vi "Auton Ramper.vi"(9 "Target Setpoint":dbl=3.01, 11 "Rate":dbl) -> (1 "Ramping":bool, 3 "Current Setpoint":dbl)   [LabVIEW 2011]
uses:
  Robot Global Data.vi
panel:
  out "crement":dbl
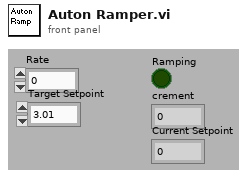
[diagram p1: front panel]
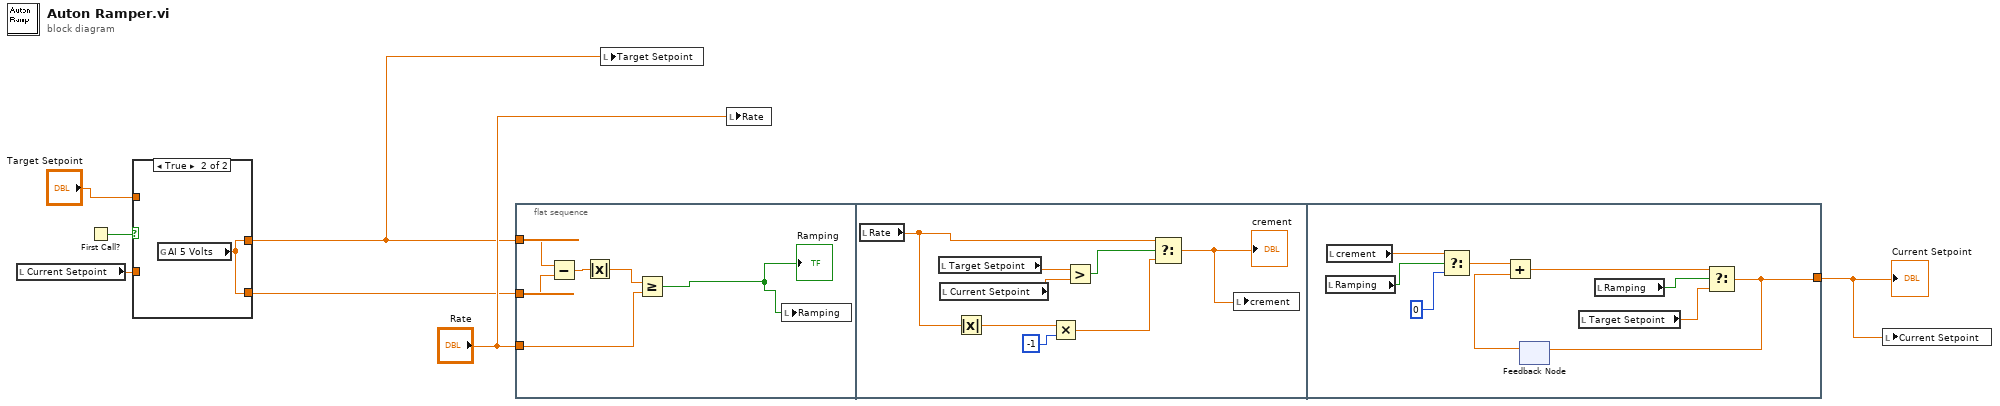
[diagram p0: block diagram]
diagram:
  n1 = local read "Current Setpoint"() -> (w4:dbl)
  n2 = First Call?() -> (First Call?: T/F=w3:bool)
  n3 = case shown="True" w3 {
    tunnel: "Target Setpoint" -> [w9 _]
    tunnel: w4 -> [w8 _]
    tunnel: [w9 w10] -> w2
    tunnel: [w8 w10] -> w1
    frame False {
    }
    frame True {
      n4 = global read "Robot Global Data.vi" "AI 5 Volts"() -> (w10:dbl)
    }
  }
  n5 = flat-sequence {
    tunnel: w2 -> [w12]
    tunnel: w1 -> [w14]
    tunnel: "Rate" -> [w13]
    tunnel: [w26] -> w6
    frame #0 {
      n6 = Subtract(x=w12, y=w14) -> (x-y=w15:dbl)
      n7 = Absolute Value(x=w15) -> (abs(x)=w16:dbl)
      n8 = Greater Or Equal?(x=w16, y=w13) -> (x >= y?=w11:bool)
      "Ramping" <- w11
      n9 = local write "Ramping"(w11) -> ()
    }
    frame #1 {
      n10 = local read "Rate"() -> (w21:dbl)
      n11 = local read "Target Setpoint"() -> (w24:dbl)
      n12 = local read "Current Setpoint"() -> (w23:dbl)
      n13 = Absolute Value(x=w21) -> (abs(x)=w20:dbl)
      n14 = Multiply(x=w20, y=-1) -> (x*y=w18:dbl)
      n15 = Greater?(x=w24, y=w23) -> (0:w22:bool)
      n16 = Select(t=w21, s=w22, f=w18) -> (s? t:f=w17:dbl)
      "crement" <- w17
      n17 = local write "crement"(w17) -> ()
    }
    frame #2 {
      n18 = local read "Ramping"() -> (w32:bool)
      n19 = local read "crement"() -> (w33:dbl)
      n20 = Select(t=w33, s=w32, f=0) -> (s? t:f=w30:dbl)
      n21 = feedback #1() -> (w27:dbl)  [unwired: 1 out]
      n22 = Add(x=w30, y=w27) -> (x+y=w29:dbl)
      n23 = local read "Target Setpoint"() -> (w28:dbl)
      n24 = local read "Ramping"() -> (w25:bool)
      n25 = Select(t=w29, s=w25, f=w28) -> (s? t:f=w26:dbl)
      n26 = feedback-in #1(w26) -> ()
    }
  }
  n27 = local write "Target Setpoint"(w2) -> ()
  n28 = local write "Rate"("Rate") -> ()
  n29 = local write "Current Setpoint"(w6) -> ()
  "Current Setpoint" <- w6
